vi "Create Delete Symbol Overlays_Properties.vi"(11 "Tree Ref":refnum<vi>) -> ()   [LabVIEW 2023]
panel:
  in  "Tree":string[](tree)
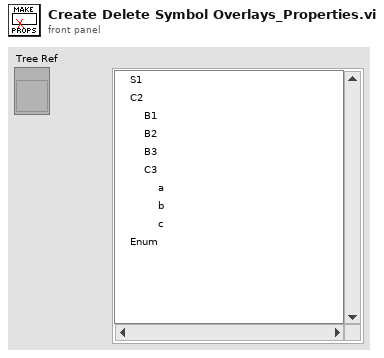
[diagram p1: front panel]
types:
  T1 = cluster{"left":i16, "top":i16, "right":i16, "bottom":i16}
  T2 = cluster{"image type":i32, "image depth":i32, "image":u8[], "mask":u8[], "colors":u32[], "Rectangle":cluster{"left":i16, "top":i16, "right":i16, "bottom":i16}}[]
  T3 = cluster{"image type":i32, "image depth":i32, "image":u8[], "mask":u8[], "colors":u32[], "Rectangle":cluster{"left":i16, "top":i16, "right":i16, "bottom":i16}}
  T4 = typedef "imagedata.ctl" = cluster{"image type":i32, "image depth":i32, "image":u8[], "mask":u8[], "colors":u32[], "Rectangle":cluster{"left":i16, "top":i16, "right":i16, "bottom":i16}}
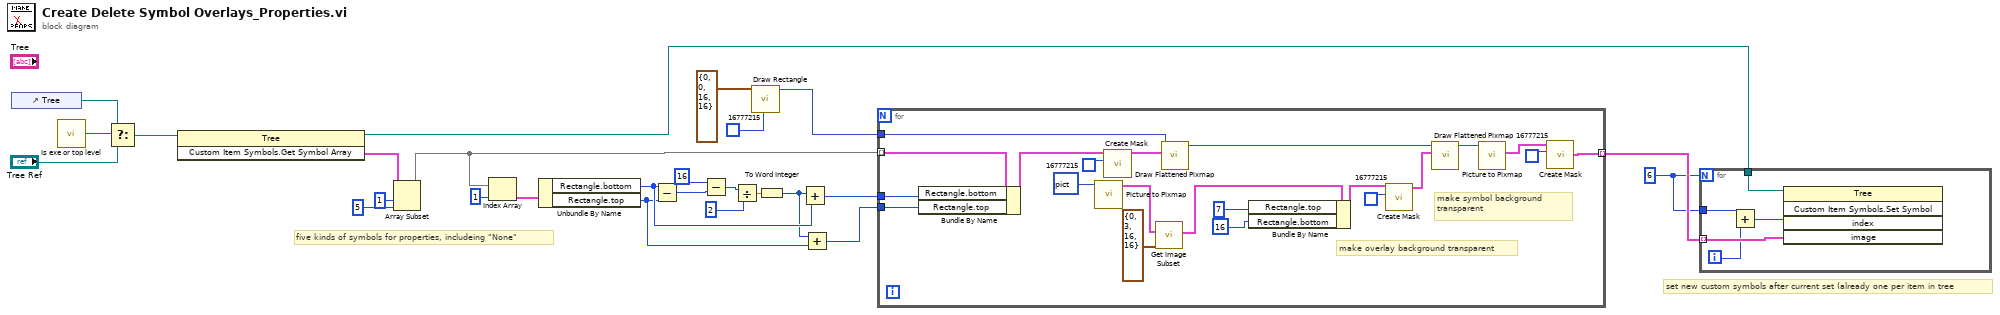
[diagram p0: block diagram]
diagram:
  w2 = 6
  # "five kinds of symbols for properties, includeing \"None\""
  # "set new custom symbols after current set (already one per item in tree"
  n1 = control-ref of="Tree"() -> (w21:refnum<vi>)
  n2 = call "Is exe or top level.vi"() -> ("Top Level?"=w22:bool)  [unwired: 5 in]
  n3 = Select(t=w21, s=w22, f="Tree Ref") -> (s? t:f=w7:refnum<vi>)
  n4 = invoke class="Tree" method="Custom Item Symbols.Get Symbol Array"(reference=w7) -> (reference out=w1:refnum<vi>, "Custom Glyphs:Get Glyph Array"=w5:T2)  [unwired: 2 in, 1 out]
  n5 = Array Subset(array=w5, index=1, length=5 ("index")) -> (w4:T2)
  n6 = Index Array(array=w4, index=1) -> (element=w15:T3)
  n7 = Unbundle By Name(w15) -> ("Rectangle.bottom"=w14:i16, "Rectangle.top"=w13:i16)
  n8 = Subtract(x=w14, y=w13) -> (x-y=w16:i16)
  n9 = Subtract(x=i16 16 ("bottom"), y=w16) -> (x-y=w18:i16)
  n10 = Divide(x=w18, y=i16 2 ("bottom")) -> (x/y=w12:dbl)
  n11 = call <vilib>:"Draw Rectangle.vi"("rect"=T1 {"left"=0, "top"=0, "right"=16, "bottom"=16}, "color(black)"=u32 16777215) -> ("new picture"=w23:picture)  [unwired: 7 in]
  n12 = To Word Integer(number=w12) -> (16bit integer=w9:i16)
  n13 = Add(x=w9, y=w14) -> (x+y=w8:i16)
  n14 = Add(x=w9, y=w13) -> (x+y=w11:i16)
  n15 = for {
    tunnel: [w27] -> w26 mode=indexing
    tunnel: w4 -> [w40] mode=indexing
    tunnel: w23 -> [w43]
    tunnel: w8 -> [w42]
    tunnel: w11 -> [w41]
    # "make symbol background transparent"
    # "make overlay background transparent"
    n16 = Bundle By Name(cluster=w40, "Rectangle.bottom"=w42, "Rectangle.top"=w41) -> (w32:T3)
    n17 = call <vilib>:"Picture to Pixmap.vi"("picture"=picture bytes[830] ("new picture")) -> ("image data"=w38:T4)  [unwired: 9 in, 1 out]
    n18 = call <vilib>:"Create Mask.vi"("Mask Color (Black)"=u32 16777215, "image data"=w32) -> ("image data"=w31:T4)  [unwired: 9 in]
    n19 = call <vilib>:"Get Image Subset.vi"("subset rect"=T1 {"left"=0, "top"=3, "right"=16, "bottom"=16}, "image data"=w38) -> ("image subset"=w37:T4)  [unwired: 4 in, 1 out]
    n20 = call <vilib>:"Draw Flattened Pixmap.vi"("image data"=w31, "picture"=w43) -> ("new picture"=w46:picture)  [unwired: 7 in]
    n21 = Bundle By Name(cluster=w37, "Rectangle.top"=i16 7 ("left"), "Rectangle.bottom"=i16 16 ("left")) -> (w36:T4)
    n22 = call <vilib>:"Create Mask.vi"("Mask Color (Black)"=u32 16777215, "image data"=w36) -> ("image data"=w45:T4)  [unwired: 9 in]
    n23 = call <vilib>:"Draw Flattened Pixmap.vi"("image data"=w45, "picture"=w46) -> ("new picture"=w30:picture)  [unwired: 7 in]
    n24 = call <vilib>:"Picture to Pixmap.vi"("picture"=w30) -> ("image data"=w29:T4)  [unwired: 9 in, 1 out]
    n25 = call <vilib>:"Create Mask.vi"("Mask Color (Black)"=u32 16777215, "image data"=w29) -> ("image data"=w27:T4)  [unwired: 9 in]
  }
  n26 = for {
    N: w2 -> [_]
    tunnel: w26 -> [w52] mode=indexing
    tunnel: w2 -> [w51]
    tunnel: w1 -> [w48]
    i -> [w50]
    n27 = Add(x=w51, y=w50) -> (x+y=w49:i32)
    n28 = invoke class="Tree" method="Custom Item Symbols.Set Symbol"(reference=w48, "index"=w49, "image"=w52) -> ()  [unwired: 2 in, 5 out]
  }
